vi "Output Enable Read Array.vi"(8 "error in":errorcluster, 11 "Cycler in":refnum<class "Cycler.lvclass">) -> (0 "error out":errorcluster, 2 "Output Enable ACT":bool[](array[boolean]), 3 "Cycler out":refnum<class "Cycler.lvclass">)   [LabVIEW 2023, in "Cycler.lvclass"]
uses:
  Cycler.lvclass
  Cycler.lvclass/Cycler.ctl
  Low Level Capabilities/Output Enable/Output Enable.lvclass
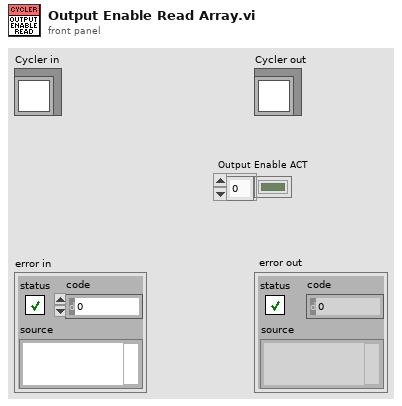
[diagram p1: front panel]
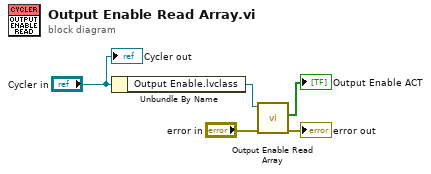
[diagram p0: block diagram]
diagram:
  n1 = Unbundle By Name("Cycler in") -> ("Output Enable.lvclass"=w5:refnum<class "Output Enable.lvclass">)
  n2 = call-dynamic "Output Enable Read Array.vi"("error in"="error in", "Output Enable in"=w5) -> ("error out"=→"error out":errorcluster, "Output Enable ACT"=→"Output Enable ACT":bool[])  [unwired: 6 in, 2 out]
  "Cycler out" <- "Cycler in"
